vi "TestRechnung.vi"() -> ()   [LabVIEW 2016]
panel:
  out "Time":dbl
  out "Numeric 2":dbl
  in  "Numeric":dbl
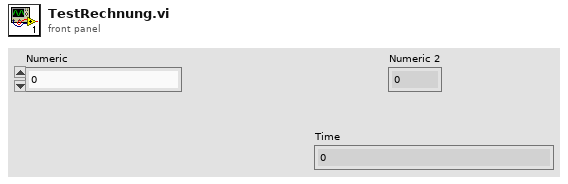
[diagram p1: front panel]
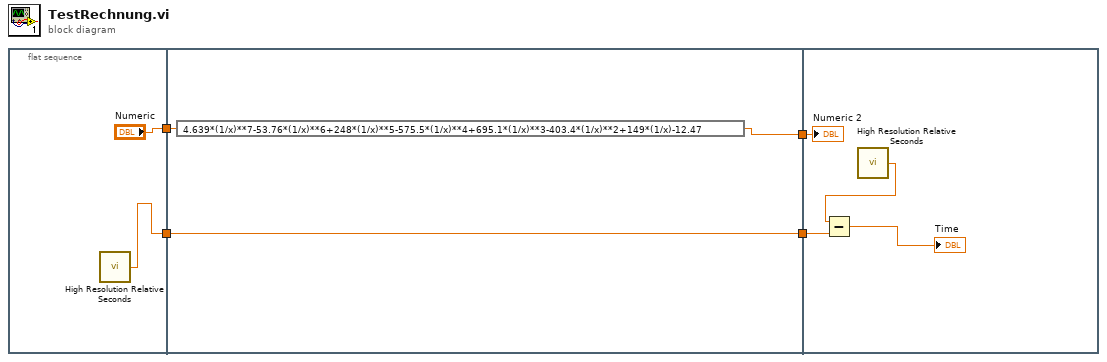
[diagram p0: block diagram]
diagram:
  n1 = flat-sequence {
    tunnel: ["Numeric"] -> w4
    tunnel: [w5] -> w1
    tunnel: w4 -> [w9]
    tunnel: [w8] -> w3
    tunnel: [w7] -> w2
    tunnel: w1 -> [w7]
    tunnel: w3 -> [w13]
    tunnel: w2 -> [w12]
    frame #0 {
      n2 = call <vilib>:"High Resolution Relative Seconds.vi"() -> ("relative seconds"=w5:dbl)
    }
    frame #1 {
      n3 = expression code="4.639*(1/x)**7-53.76*(1/x)**6+248*(1/x)**5-575.5*(1/x)**4+695.1*(1/x)**3-403.4*(1/x)**2+149*(1/x)-12.47"(w9) -> (w8:dbl)
    }
    frame #2 {
      n4 = call <vilib>:"High Resolution Relative Seconds.vi"() -> ("relative seconds"=w10:dbl)
      n5 = Subtract(x=w10, y=w12) -> (x-y=→"Time":dbl)
      "Numeric 2" <- w13
    }
  }
